vi "RGB (SubVI).vi"(1 "Color":enum16{"R", "AZ", "AM", "N", "V", "B", "C"}(ring)) -> (0 "Color":u32(colorbox))   [LabVIEW 2013]
panel:
  in  "Color":T1(ring)
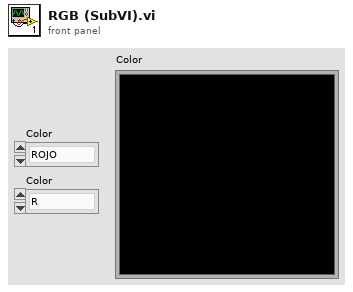
[diagram p1: front panel]
types:
  T1 = enum16{"ROJO", "AZUL", "AMARILLO", "NEGRO", "VERDE", "BLANCO"}
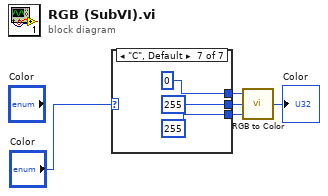
[diagram p0: block diagram]
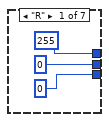
[diagram p2: hidden frame]
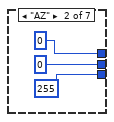
[diagram p3: hidden frame]
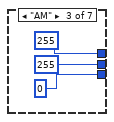
[diagram p4: hidden frame]
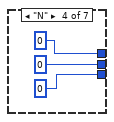
[diagram p5: hidden frame]
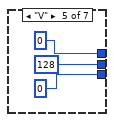
[diagram p6: hidden frame]
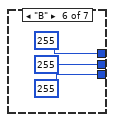
[diagram p7: hidden frame]
diagram:
  n1 = case shown="\"C\", Default" "Color" {
    tunnel: [0 0 255 0 128 255 255] -> w5
    tunnel: [255 0 255 0 0 255 0] -> w4
    tunnel: [0 255 0 0 0 255 255] -> w3
    frame "R" {
    }
    frame "AZ" {
    }
    frame "AM" {
    }
    frame "N" {
    }
    frame "V" {
    }
    frame "B" {
    }
    frame "C", Default {
    }
  }
  n2 = call <vilib>:"RGB to Color.vi"("B"=w3, "G"=w5, "R"=w4) -> ("Color"=→"Color":u32)
